vi "Chaining Promises With Unexpected Deletion.vi"(8 "error in (no error)":errorcluster) -> (0 "error out":errorcluster)   [LabVIEW 2017, in "Unit Tests.lvlib"]
uses:
  Unit Tests.lvlib
  d5346042-4ec6-404b-8c5f-dbc4908b2214.vi
  76facaf0-d6b8-4456-945a-d490993a15ec.vi
  c8fde1cb-f932-48ba-af77-c4f1b9334ea4.vi
  7457912a-0468-4450-95f8-5e7f7be31632.vi
  ed79e3ae-d641-450c-a703-6c473cd6614a.vi
  Promise Future/Promise/Promise.lvclass
  E:/Promise/Promise Future/Future/Future.lvclass
  Promise Future/Future/Write Future.vi
  Promise Future/Future/Read Value.vi
  <vilib>/addons/_JKI Toolkits/Caraya/classes/Test/Test.lvclass
  <vilib>/addons/_JKI Toolkits/Caraya/classes/Assert/Assert.lvclass
  Promise Future/Future/Future.lvclass
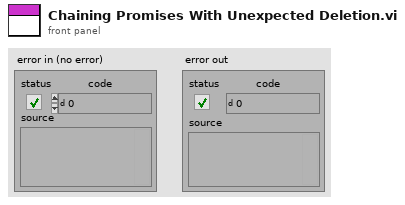
[diagram p1: front panel]
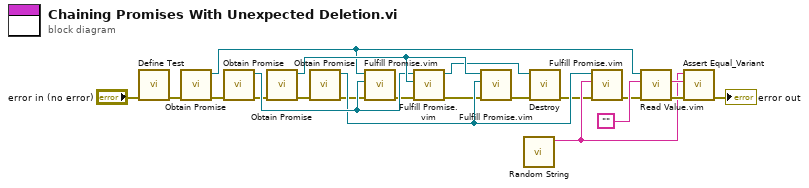
[diagram p0: block diagram]
diagram:
  n1 = call <vilib>:"Define Test.vi"("error in (no error)"="error in (no error)") -> ("error out"=w2:errorcluster)  [unwired: 10 in]
  n2 = call "Obtain Promise.vi"("error in (no error)"=w2) -> ("error out"=w12:errorcluster, "Promise out"=w3:refnum<class "Promise.lvclass">)  [unwired: 8 in, 1 out]
  n3 = call "Obtain Promise.vi"("error in (no error)"=w12) -> ("error out"=w11:errorcluster, "Promise out"=w15:refnum<class "Promise.lvclass">)  [unwired: 8 in, 1 out]
  n4 = call "Obtain Promise.vi"("error in (no error)"=w11) -> ("error out"=w10:errorcluster, "Promise out"=w16:refnum<class "Promise.lvclass">)  [unwired: 8 in, 1 out]
  n5 = call "Obtain Promise.vi"("error in (no error)"=w10) -> ("error out"=w4:errorcluster, "Promise out"=w14:refnum<class "Promise.lvclass">)  [unwired: 8 in, 1 out]
  n6 = call "Fulfill Promise.vim"("error in (no error)"=w4, "Value"=w15, "Promise in"=w3) -> ("error out"=w9:errorcluster)  [unwired: 7 in, 1 out]
  n7 = call "Fulfill Promise.vim"("error in (no error)"=w9, "Value"=w16, "Promise in"=w15) -> ("error out"=w8:errorcluster, "Promise out"=w7:refnum<class "Promise.lvclass">)  [unwired: 7 in]
  n8 = call "Fulfill Promise.vim"("error in (no error)"=w8, "Value"=w14, "Promise in"=w16) -> ("error out"=w6:errorcluster)  [unwired: 7 in, 1 out]
  n9 = call "Random String.vi"() -> ("string"=w13:string)  [unwired: 11 in]
  n10 = call "Destroy.vi"("error in (no error)"=w6, "Future in"=w7) -> ("error out"=w5:errorcluster)  [unwired: 9 in]
  n11 = call "Fulfill Promise.vim"("error in (no error)"=w5, "Value"=w13, "Promise in"=w14) -> ("error out"=w1:errorcluster)  [unwired: 7 in, 1 out]
  n12 = call "Read Value.vim"("error in (no error)"=w1, "Default Value"="", "Future in"=w3) -> ("error out"=w19:errorcluster, "Value"=w17:string)  [unwired: 5 in, 2 out]
  n13 = call <vilib>:"Assert Equal_Variant.vi"("error in (no error)"=w19, "Y"=w17, "X"=w13) -> ("error out"=→"error out":errorcluster)  [unwired: 8 in]
